vi "Average xy graphs.vi"(1 "end":dbl, 2 "step":dbl, 3 "start":dbl, 4 "IGA":cluster{dbl[], dbl[]}[](graph)) -> (0 "IGA average":cluster{dbl[], dbl[]}(graph))   [LabVIEW 2010]
uses:
  <vilib>/Analysis/NI_AALBase.lvlib
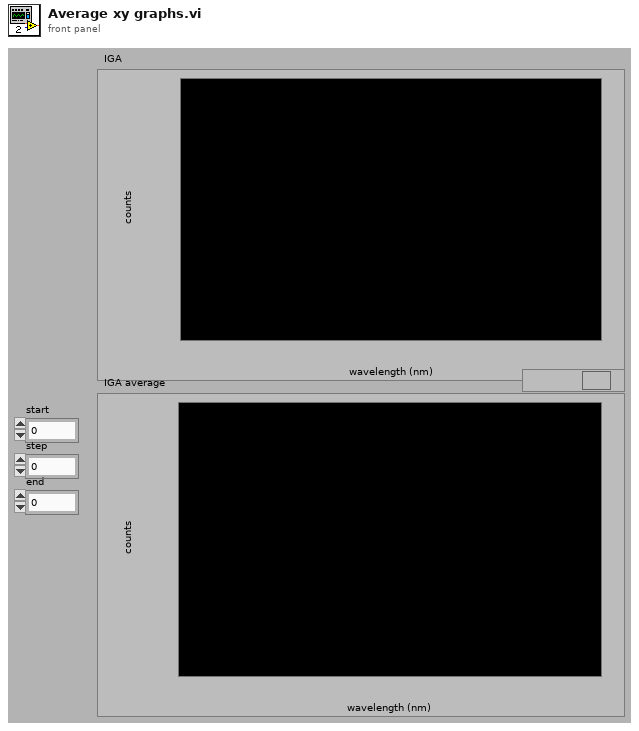
[diagram p1: front panel]
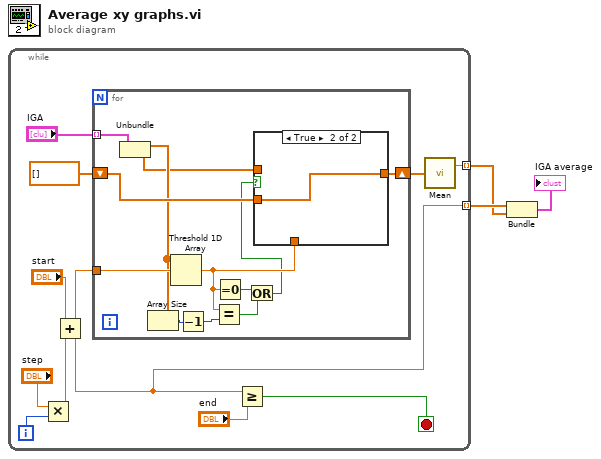
[diagram p0: block diagram]
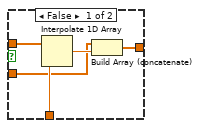
[diagram p2: hidden frame]
diagram:
  n1 = while {
    tunnel: [w7] -> w1 mode=indexing
    tunnel: [w5] -> w3 mode=indexing
    i -> [w13]
    stop <- w8 stop-if-true
    n2 = Multiply(x="step", y=w13) -> (x*y=w10:dbl)
    n3 = Add(x="start", y=w10) -> (x+y=w5:dbl)
    n4 = for {
      tunnel: "IGA" -> [w26] mode=indexing
      shift-right: [w25] -> w4
      shift-left: dbl[] [] -> [w24]
      tunnel: w5 -> [w23]
      n5 = Unbundle(w26) -> (w22:dbl[], w17:dbl[])
      n6 = Array Size(array=w22) -> (size(s)=w16:i32)
      n7 = Threshold 1D Array(2:w23, 3:w22) -> (0:w20:dbl)  [unwired: 1 in]
      n8 = Decrement(x=w16) -> (x-1=w15:i32)
      n9 = Equal?(x=w20, y=w15) -> (x = y?=w19:bool)
      n10 = Equal To 0?(x=w20) -> (x = 0?=w21:bool)
      n11 = Or(x=w21, y=w19) -> (x .or. y?=w18:bool)
      n12 = case shown="True" w18 {
        tunnel: [w29 w32] -> w25
        tunnel: w20 -> [w31 _]
        tunnel: w17 -> [w30 _]
        tunnel: w24 -> [w27 w32]
        frame False {
          n13 = Interpolate 1D Array(1:w31, 2:w30) -> (0:w28:dbl)
          n14 = Build Array (concatenate)(w27, w28) -> (w29:dbl[])
        }
        frame True {
        }
      }
    }
    n15 = Greater Or Equal?(x=w5, y="end") -> (x >= y?=w8:bool)
    n16 = call <vilib>:"Mean.vi"("X"=w4) -> ("mean"=w7:dbl)  [unwired: 1 out]
  }
  n17 = Bundle(w3, w1) -> (→"IGA average":cluster{dbl[], dbl[]})  [unwired: 1 in]
